vi "Read Handle.vi"(8 "Error In":errorcluster, 11 "Known Host In":refnum<class "Known Host.lvclass">) -> (0 "Error Out":errorcluster, 2 "Handle":u64, 3 "Known Host Out":refnum<class "Known Host.lvclass">)   [LabVIEW 2018, in "Toolkit.lvlib" / "Known Host.lvclass"]
uses:
  Known Host.lvclass
  Known Host.lvclass/Known Host.ctl
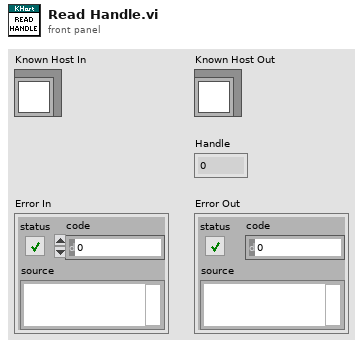
[diagram p1: front panel]
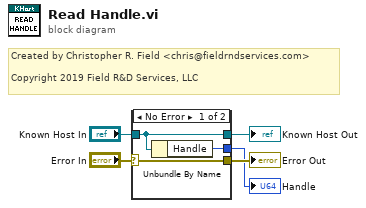
[diagram p0: block diagram]
diagram:
  # "Created by Christopher R. Field <chris@fieldrndservices.com>\n\nCopyright 2019 Field R&D Services, LLC"
  n1 = case shown="No Error" "Error In" {
    selector: "Error In" -> [w7 w10]
    tunnel: "Known Host In" -> [w8 w9]
    tunnel: [w8 w9] -> w3
    tunnel: [w7 w10] -> w2
    tunnel: [w6 _] -> w1
    frame No Error {
      n2 = Unbundle By Name(w8) -> ("Handle"=w6:u64)
    }
    frame Error {
    }
  }
  "Known Host Out" <- w3
  "Error Out" <- w2
  "Handle" <- w1
